vi "previousTrack.vi"(8 "error in (no error)":errorcluster, 11 "Player in":refnum<class "Player.lvclass">) -> (0 "error out":errorcluster, 2 "Song":string, 3 "Player out":refnum<class "Player.lvclass">)   [LabVIEW 2018, in "Player.lvclass"]
uses:
  Player.lvclass
  Player.lvclass/Player.ctl
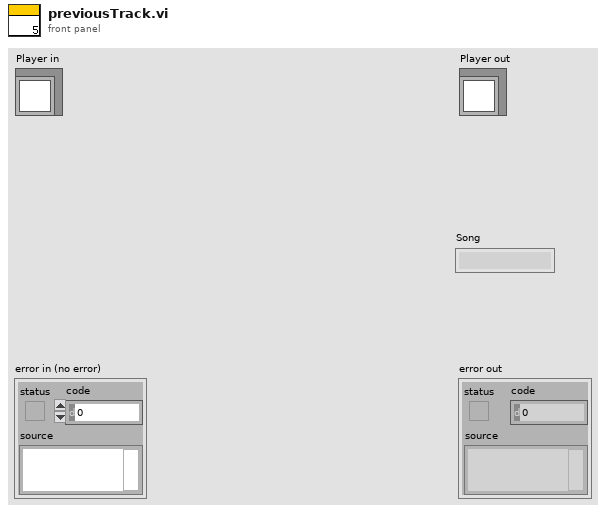
[diagram p1: front panel]
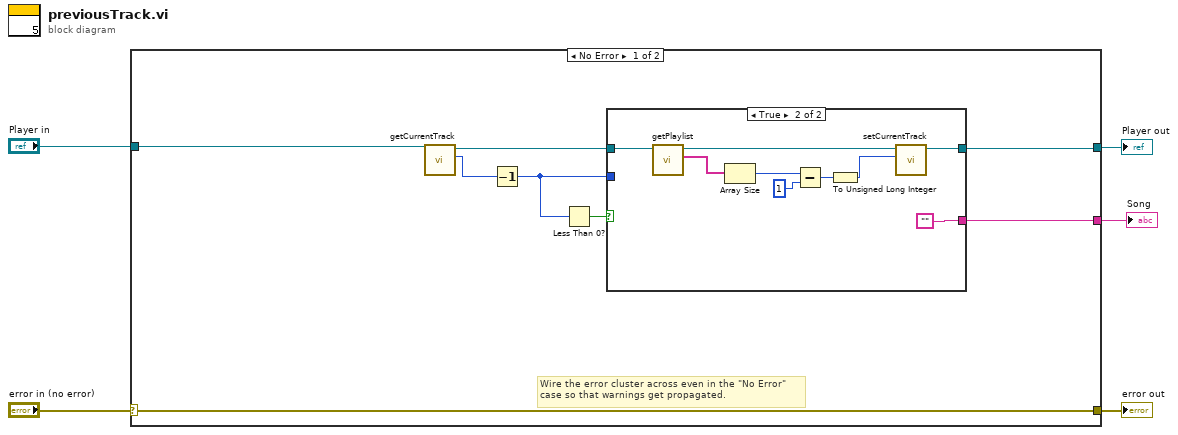
[diagram p0: block diagram]
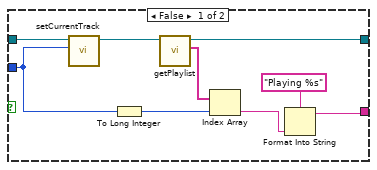
[diagram p2: hidden frame]
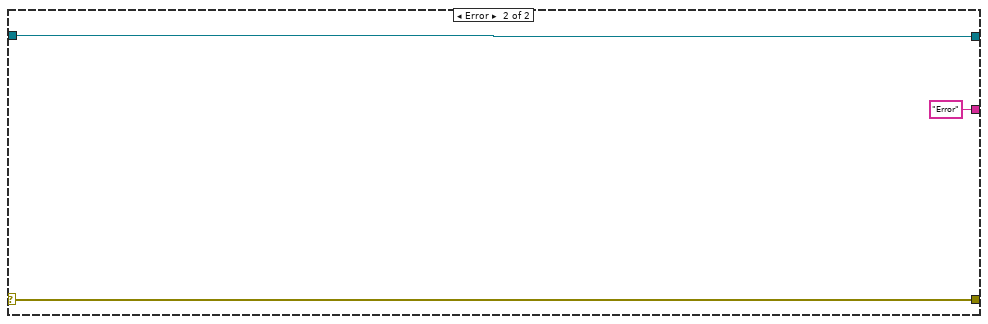
[diagram p3: hidden frame]
diagram:
  n1 = case shown="No Error" "error in (no error)" {
    selector: "error in (no error)" -> [w13 w34]
    tunnel: [w13 w34] -> w4
    tunnel: [w9 w33] -> w2
    tunnel: "Player in" -> [w6 w33]
    tunnel: [w8 "Error"] -> w1
    frame No Error {
      # "Wire the error cluster across even in the \"No Error\"\ncase so that warnings get propagated."
      n2 = call "getCurrentTrack.vi"("Player in"=w6) -> ("currentTrack"=w10:u32, "Player out"=w11:refnum<class "Player.lvclass">)  [unwired: 8 in, 1 out]
      n3 = Decrement(x=w10) -> (x-1=w7:u32)
      n4 = Less Than 0?(x=w7) -> (x < 0?=w12:bool)
      n5 = case shown="True" w12 {
        tunnel: w11 -> [w22 w26]
        tunnel: [w20 w31] -> w9
        tunnel: [w16 ""] -> w8
        tunnel: w7 -> [w18 _]
        frame False {
          n6 = call "setCurrentTrack.vi"("currentTrack"=w18, "Player in"=w22) -> ("Player out"=w21:refnum<class "Player.lvclass">)  [unwired: 8 in, 1 out]
          n7 = To Long Integer(number=w18) -> (32bit integer=w17:i32)
          n8 = call "getPlaylist.vi"("Player in"=w21) -> ("Playlist"=w19:string[], "Player out"=w20:refnum<class "Player.lvclass">)  [unwired: 8 in, 1 out]
          n9 = Index Array(array=w19, index=w17) -> (element=w15:string)
          n10 = Format Into String(format string="Playing %s", w15) -> (resulting string=w16:string)  [unwired: 2 in, 1 out]
        }
        frame True {
          n11 = call "getPlaylist.vi"("Player in"=w26) -> ("Playlist"=w29:string[], "Player out"=w25:refnum<class "Player.lvclass">)  [unwired: 8 in, 1 out]
          n12 = Array Size(array=w29) -> (size(s)=w28:i32)
          n13 = Subtract(x=w28, y=1) -> (x-y=w24:i32)
          n14 = To Unsigned Long Integer(number=w24) -> (unsigned 32bit integer=w23:u32)
          n15 = call "setCurrentTrack.vi"("currentTrack"=w23, "Player in"=w25) -> ("Player out"=w31:refnum<class "Player.lvclass">)  [unwired: 8 in, 1 out]
        }
      }
    }
    frame Error {
    }
  }
  "error out" <- w4
  "Player out" <- w2
  "Song" <- w1
